vi "pr650_main.vi"() -> ()   [LabVIEW 2010]
panel:
  out "concatenated string":string
  out "timestamp":string
  in  "save to file?":bool
  in  "save path":path
  in  "Repeat cycles":dbl
  out "Card Batt":bool
  out "Main Batt":bool
  out "Comm OK":bool
  in  "Connect":bool
  in  "Execute Custom command":bool
  out "VISA resource":refnum<visa-resource-name>
  out "Last measurement":cluster{"Y":dbl[], "Y":dbl[]}[](graph)
  out "data transfer":bool
  out "array":dbl[][](array[numeric])
  out "stopping":bool
  in  "Go!":bool
  in  "custom command":string
  out "read buffer":string
  out "bytes at port":u32
  out "return count":u32
  in  "stop":bool
  out "error out":errorcluster
  in  "PR650 COM port":refnum<visa-resource-name>
  # "Connection"
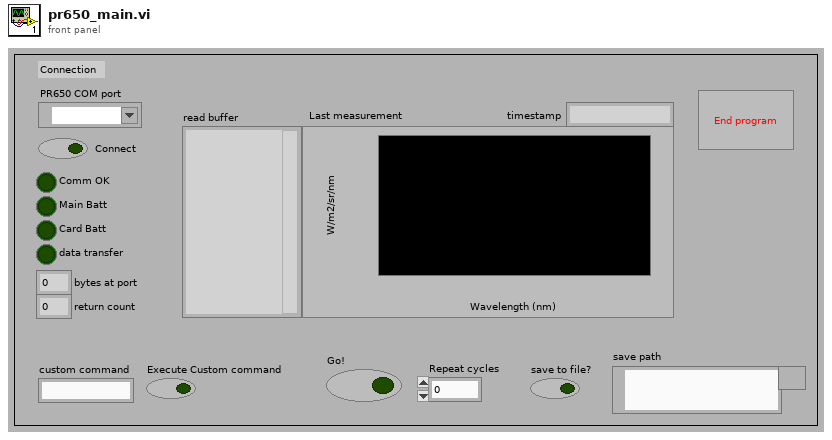
[diagram p1: front panel]
types:
  T1 = enum16{"open", "replace", "create", "open or create", "replace or create", "replace or create with confirmation"}
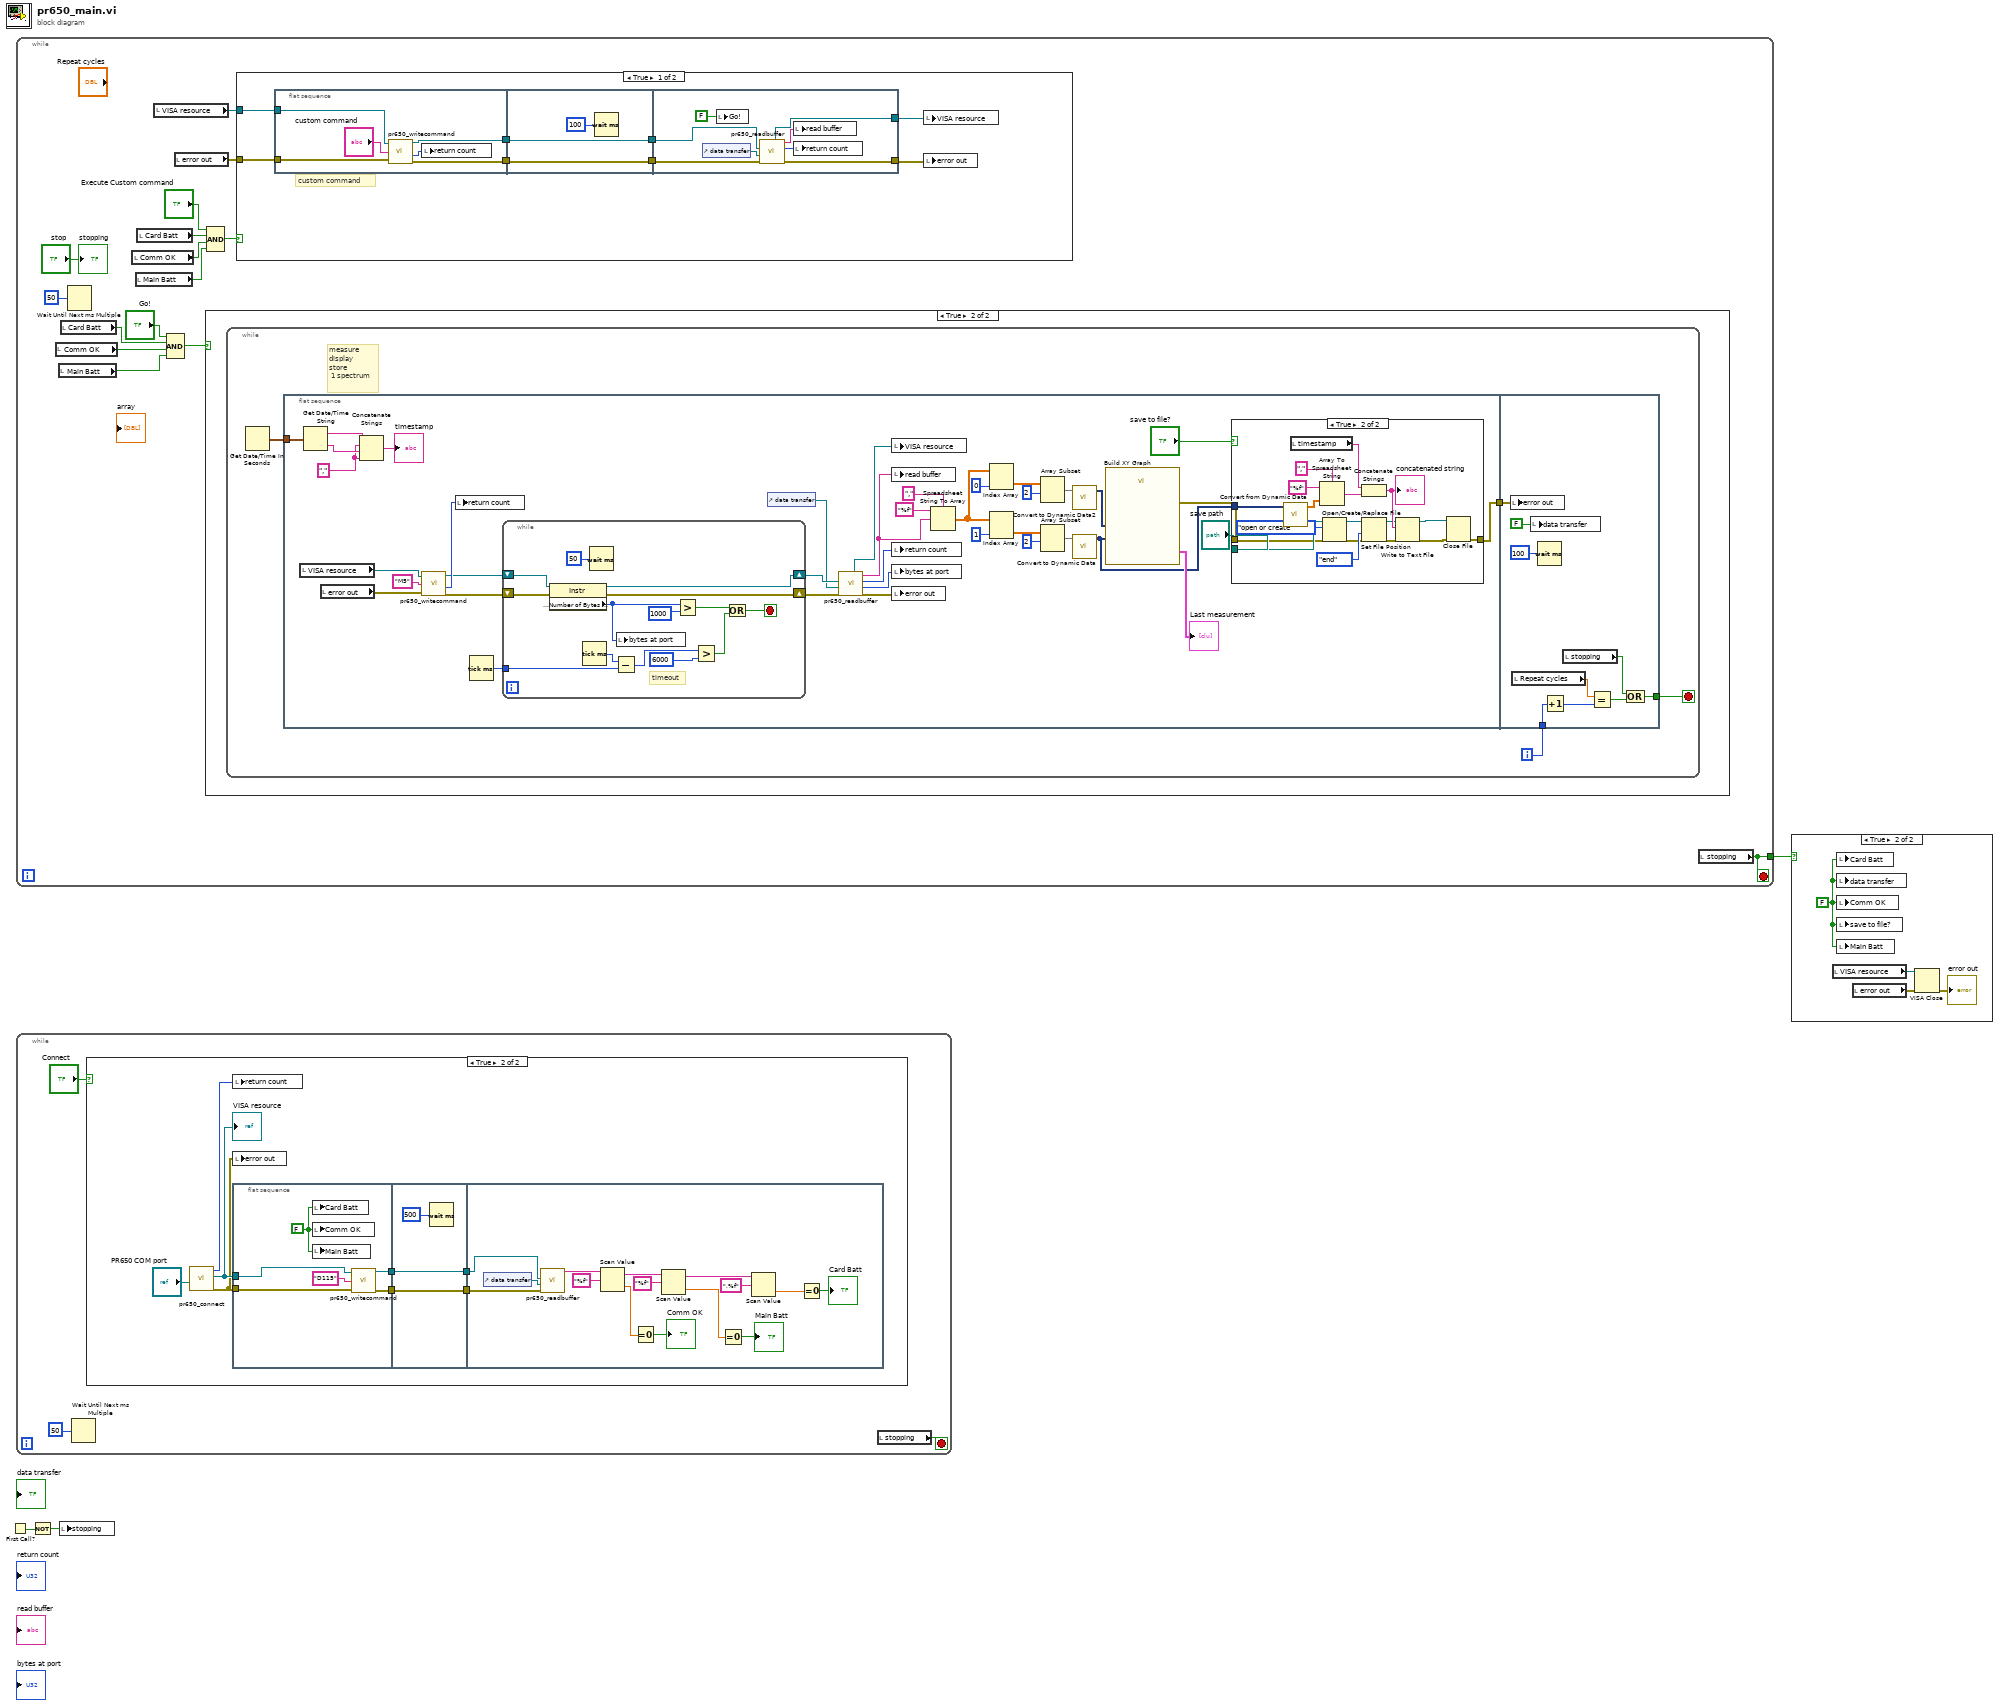
[diagram p0: block diagram]
diagram:
  n1 = First Call?() -> (First Call?: T/F=w3:bool)
  n2 = while {
    tunnel: [w16] -> w1
    stop <- w16 stop-if-true
    n3 = local read "Comm OK"() -> (w10:bool)
    n4 = local read "Main Batt"() -> (w9:bool)
    n5 = local read "Card Batt"() -> (w11:bool)
    n6 = Wait Until Next ms Multiple(millisecond multiple=u32 50) -> ()  [unwired: 1 out]
    n7 = local read "Comm OK"() -> (w7:bool)
    n8 = local read "Main Batt"() -> (w8:bool)
    n9 = local read "Card Batt"() -> (w6:bool)
    n10 = local read "VISA resource"() -> (w13:refnum<visa-resource-name>)
    n11 = Compound Arithmetic op=AND("Go!", w11, w10, w9) -> (w15:bool)
    n12 = local read "error out"() -> (w12:errorcluster)
    n13 = case shown="True" w15 {
      frame False {
      }
      frame True {
        n14 = while {
          i -> [w47]
          stop <- w46 stop-if-true
          # "measure\ndisplay\nstore\n 1 spectrum"
          n15 = Get Date/Time In Seconds() -> (seconds since 1Jan1904=w44:timestamp)
          n16 = flat-sequence {
            tunnel: [w55] -> w45
            tunnel: w44 -> [w52]
            tunnel: w47 -> [w125]
            tunnel: [w124] -> w46
            tunnel: w45 -> [w122]
            frame #0 {
              w48 = ","
              n17 = local read "VISA resource"() -> (w78:refnum<visa-resource-name>)
              n18 = Get Date/Time String(seconds (now)=w52) -> (date string=w51:string, time string=w49:string)  [unwired: 2 in]
              n19 = local read "error out"() -> (w77:errorcluster)
              n20 = Concatenate Strings(w51, w48, w49, w48) -> (→"timestamp":string)
              n21 = call "pr650_writecommand.vi"("error in"=w77, "write buffer"="M5" ("string"), "VISA resource name in"=w78) -> ("error out"=w58:errorcluster, "return count"=w80:u32, "VISA resource name out"=w59:refnum<visa-resource-name>)  [unwired: 1 in]
              n22 = local write "return count"(w80) -> ()
              n23 = Tick Count (ms)() -> (millisecond timer value=w76:u32)
              n24 = while {
                shift-right: [w118] -> w84
                shift-left: w59 -> [w116]
                shift-right: [w117] -> w85
                shift-left: w58 -> [w105]
                tunnel: w76 -> [w109]
                stop <- w111 stop-if-true
                # "timeout"
                n25 = property class="Instr"(reference=w116, error in=w105) -> (reference out=w118:refnum<visa-resource-name>, error out=w117:errorcluster, "Serial Settings:Number of Bytes at Serial Port"=w115:u32)
                n26 = Tick Count (ms)() -> (millisecond timer value=w110:u32)
                n27 = Wait (ms)(milliseconds to wait=u32 50) -> ()  [unwired: 1 out]
                n28 = Subtract(x=w110, y=w109) -> (x-y=w108:u32)
                n29 = local write "bytes at port"(w115) -> ()
                n30 = Greater?(x=w115, y=u32 1000) -> (0:w113:bool)
                n31 = Greater?(x=w108, y=u32 6000) -> (0:w106:bool)
                n32 = Or(x=w113, y=w106) -> (x .or. y?=w111:bool)
              }
              n33 = control-ref of="data transfer"() -> (w73:refnum<vi>)
              n34 = call "pr650_readbuffer.vi"("error in (no error)"=w85, "ref"=w73, "reference"=w84) -> ("error out"=w83:errorcluster, "bytes at port"=w70:u32, "return count"=w72:u32, "read buffer"=w71:string, "VISA resource name out"=w82:refnum<visa-resource-name>)  [unwired: 2 in]
              n35 = local write "VISA resource"(w82) -> ()
              n36 = local write "read buffer"(w71) -> ()
              n37 = local write "return count"(w72) -> ()
              n38 = local write "bytes at port"(w70) -> ()
              n39 = local write "error out"(w83) -> ()
              n40 = Spreadsheet String To Array(delimiter (Tab)=",", format string="%f", spreadsheet string=w71) -> (array=w81:dbl[][])  [unwired: 1 in]
              n41 = Index Array(array=w81, index (col)=0 ("index")) -> (element=w65:dbl[])  [unwired: 1 in]
              n42 = Index Array(array=w81, index (col)=1 ("index")) -> (element=w62:dbl[])  [unwired: 1 in]
              n43 = Array Subset(array=w65, index=2) -> (w68:dbl[])  [unwired: 1 in]
              n44 = Array Subset(array=w62, index=2) -> (w67:dbl[])  [unwired: 1 in]
              n45 = call "Convert to Dynamic Data2"("Array"=w68) -> ("Dynamic Data Type"=w69:dynamicdata)  [unwired: 3 in]
              n46 = call "Convert to Dynamic Data"("Array"=w67) -> ("Dynamic Data Type"=w57:dynamicdata)  [unwired: 3 in]
              n47 = call "Build XY Graph"("Y Input"=w57, "X Input"=w69) -> ("error out"=w56:errorcluster, "XY Graph"=→"Last measurement":cluster{"Y":dbl[], "Y":dbl[]}[])  [unwired: 3 in, 5 out]
              n48 = case shown="True" "save to file?" {
                tunnel: w57 -> [_ w104]
                tunnel: w56 -> [w86 w93]
                tunnel: [w86 w88] -> w55
                tunnel: "save path" -> [_ w94]
                frame False {
                }
                frame True {
                  n49 = call "Convert from Dynamic Data"("Dynamic Data Type"=w104) -> ("Array"=w103:dbl[])  [unwired: 3 in]
                  n50 = local read "timestamp"() -> (w101:string)
                  n51 = Array To Spreadsheet String(delimiter (Tab)=",", array=w103, 3:"%f" ("format string")) -> (spreadsheet string=w100:string)
                  n52 = Open/Create/Replace File(file path (use dialog)=w94, error in=w93, operation (0:open)=T1."open or create") -> (refnum out=w91:refnum<file>, error out=w92:errorcluster)  [unwired: 3 in, 1 out]
                  n53 = Concatenate Strings(w101, w100) -> (w98:string)
                  "concatenated string" <- w98
                  n54 = Set File Position(refnum=w91, from (0:start)=enum16{"start", "end", "current"}."end", error in=w92) -> (refnum out=w97:refnum<file>, error out=w96:errorcluster)  [unwired: 1 in]
                  n55 = Write to Text File(file (use dialog)=w97, text=w98, error in=w96) -> (refnum out=w90:refnum<file>, error out=w89:errorcluster)  [unwired: 1 in, 1 out]
                  n56 = Close File(refnum=w90, error in=w89) -> (error out=w88:errorcluster)  [unwired: 1 out]
                }
              }
            }
            frame #1 {
              n57 = local write "error out"(w122) -> ()
              n58 = local read "Repeat cycles"() -> (w123:dbl)
              n59 = local write "data transfer"(FALSE) -> ()
              n60 = Wait (ms)(milliseconds to wait=u32 100) -> ()  [unwired: 1 out]
              n61 = Increment(x=w125) -> (x+1=w119:i32)
              n62 = local read "stopping"() -> (w126:bool)
              n63 = Equal?(x=w123, y=w119) -> (x = y?=w127:bool)
              n64 = Compound Arithmetic op=OR(w126, w127) -> (w124:bool)
            }
          }
        }
      }
    }
    n65 = Compound Arithmetic op=AND("Execute Custom command", w6, w7, w8) -> (w4:bool)
    n66 = case shown="True" w4 {
      tunnel: w13 -> [w20 _]
      tunnel: w12 -> [w19 _]
      frame True {
        # "custom command"
        n67 = flat-sequence {
          tunnel: [w31] -> w26
          tunnel: [w30] -> w25
          tunnel: w20 -> [w28]
          tunnel: w19 -> [w27]
          tunnel: w26 -> [w34]
          tunnel: w25 -> [w33]
          tunnel: [w34] -> w24
          tunnel: [w33] -> w23
          tunnel: [w43] -> w21
          tunnel: [w42] -> w22
          tunnel: w24 -> [w39]
          tunnel: w23 -> [w38]
          frame #0 {
            n68 = call "pr650_writecommand.vi"("error in"=w27, "write buffer"="custom command", "VISA resource name in"=w28) -> ("error out"=w30:errorcluster, "return count"=w29:u32, "VISA resource name out"=w31:refnum<visa-resource-name>)  [unwired: 1 in]
            n69 = local write "return count"(w29) -> ()
          }
          frame #1 {
            n70 = Wait (ms)(milliseconds to wait=u32 100) -> ()  [unwired: 1 out]
          }
          frame #2 {
            n71 = control-ref of="data transfer"() -> (w36:refnum<vi>)
            n72 = local write "Go!"(FALSE ("function1")) -> ()
            n73 = call "pr650_readbuffer.vi"("error in (no error)"=w38, "ref"=w36, "reference"=w39) -> ("error out"=w43:errorcluster, "return count"=w40:u32, "read buffer"=w41:string, "VISA resource name out"=w42:refnum<visa-resource-name>)  [unwired: 2 in, 1 out]
            n74 = local write "read buffer"(w41) -> ()
            n75 = local write "return count"(w40) -> ()
          }
        }
        n76 = local write "VISA resource"(w22) -> ()
        n77 = local write "error out"(w21) -> ()
      }
      frame False {
      }
    }
    n78 = local read "stopping"() -> (w16:bool)
    "stopping" <- "stop"
  }
  n79 = while {
    stop <- w129 stop-if-true
    n80 = Wait Until Next ms Multiple(millisecond multiple=u32 50) -> ()  [unwired: 1 out]
    n81 = case shown="True" "Connect" {
      frame False {
      }
      frame True {
        n82 = call "pr650_connect.vi"("PR650 COM port"="PR650 COM port") -> ("error out"=w135:errorcluster, "VISA resource name out"=w136:refnum<visa-resource-name>, "return count"=w137:u32)  [unwired: 4 in]
        "VISA resource" <- w136
        n83 = local write "return count"(w137) -> ()
        n84 = local write "error out"(w135) -> ()
        n85 = flat-sequence {
          tunnel: w136 -> [w143]
          tunnel: w135 -> [w142]
          tunnel: [w141] -> w133
          tunnel: [w140] -> w132
          tunnel: [w146] -> w134
          tunnel: w133 -> [w146]
          tunnel: w132 -> [w145]
          tunnel: [w145] -> w131
          tunnel: w134 -> [w161]
          tunnel: w131 -> [w160]
          frame #0 {
            w139 = FALSE
            n86 = local write "Card Batt"(w139) -> ()
            n87 = local write "Comm OK"(w139) -> ()
            n88 = local write "Main Batt"(w139) -> ()
            n89 = call "pr650_writecommand.vi"("error in"=w142, "write buffer"="D115" ("string"), "VISA resource name in"=w143) -> ("error out"=w140:errorcluster, "VISA resource name out"=w141:refnum<visa-resource-name>)  [unwired: 1 in, 1 out]
          }
          frame #1 {
            n90 = Wait (ms)(milliseconds to wait=u32 500) -> ()  [unwired: 1 out]
          }
          frame #2 {
            n91 = control-ref of="data transfer"() -> (w162:refnum<vi>)
            n92 = call "pr650_readbuffer.vi"("error in (no error)"=w160, "ref"=w162, "reference"=w161) -> ("read buffer"=w159:string)  [unwired: 2 in, 4 out]
            n93 = Scan Value(string=w159, format string="%f") -> (output string=w156:string, value=w157:dbl)  [unwired: 1 in]
            n94 = Equal To 0?(x=w157) -> (x = 0?=→"Comm OK":bool)
            n95 = Scan Value(string=w156, format string="%f") -> (output string=w153:string, value=w151:dbl)  [unwired: 1 in]
            n96 = Equal To 0?(x=w151) -> (x = 0?=→"Main Batt":bool)
            n97 = Scan Value(string=w153, format string=",%f") -> (value=w148:dbl)  [unwired: 1 in, 1 out]
            n98 = Equal To 0?(x=w148) -> (x = 0?=→"Card Batt":bool)
          }
        }
      }
    }
    n99 = local read "stopping"() -> (w129:bool)
  }
  n100 = Not(x=w3) -> (.not. x?=w2:bool)
  n101 = local write "stopping"(w2) -> ()
  n102 = case shown="True" w1 {
    frame False {
    }
    frame True {
      w163 = FALSE
      n103 = local read "VISA resource"() -> (w165:refnum<visa-resource-name>)
      n104 = local write "Card Batt"(w163) -> ()
      n105 = local write "data transfer"(w163) -> ()
      n106 = local write "Comm OK"(w163) -> ()
      n107 = local write "save to file?"(w163) -> ()
      n108 = local write "Main Batt"(w163) -> ()
      n109 = local read "error out"() -> (w164:errorcluster)
      n110 = VISA Close(VISA resource name=w165, error in (no error)=w164) -> (error out=→"error out":errorcluster)
    }
  }
